vi "getDependencyDir.vi"() -> (3 "Dependency Directory":path)   [LabVIEW 2016]
panel:
  # "Returns the path to the current dependency directory \nof the project"
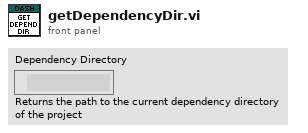
[diagram p1: front panel]
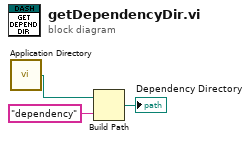
[diagram p0: block diagram]
diagram:
  n1 = call <vilib>:"Application Directory.vi"() -> ("Application Directory"=w1:path)
  n2 = Build Path(base path=w1, name or relative path="dependency") -> (appended path=→"Dependency Directory":path)
